vi "libssh2_trace.vi"(8 "error in (no error)":errorcluster, 10 "bitmask":i32(ring) items=["LIBSSH2_TRACE_TRANS"=2, "LIBSSH2_TRACE_KEX"=4, "LIBSSH2_TRACE_AUTH"=8, "LIBSSH2_TRACE_CONN"=16, "LIBSSH2_TRACE_SCP"=32, "LIBSSH2_TRACE_SFTP"=64, "LIBSSH2_TRACE_ERROR"=128, "LIBSSH2_TRACE_PUBLICKEY"=256, "LIBSSH2_TRACE_SOCKET"=512], 11 "session":T1) -> (0 "error out":errorcluster)   [LabVIEW 2017, in "libssh2.lvlib"]
doc: "Set the trace flags for libssh2."
uses:
  libssh2.lvlib
  Session Refnum.ctl
  Not A Session.vi
  <vilib>/Utility/error.llb/Error Cluster From Error Code.vi
  Global Settings.vi
  Read Session Refnum.vi
  <vilib>/Utility/semaphor.llb/Acquire Semaphore.vi
  <vilib>/Utility/semaphor.llb/Release Semaphore.vi
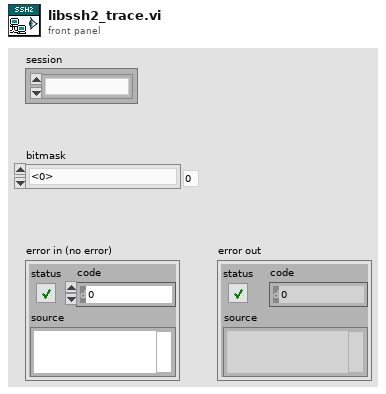
[diagram p1: front panel]
types:
  T1 = typedef "libssh2.lvlib/Session Refnum.ctl" = refnum<k1>
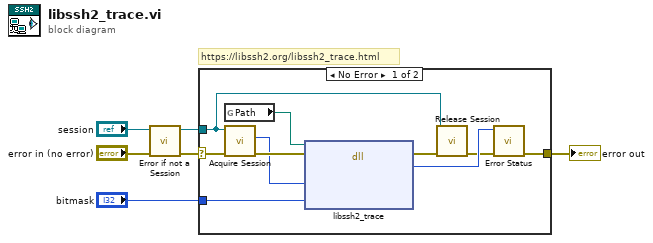
[diagram p0: block diagram]
diagram:
  # "https://libssh2.org/libssh2_trace.html"
  n1 = call "Error if not a Session.vi"("error in (no error)"="error in (no error)", "session"="session") -> ("error out"=w3:errorcluster, "session out"=w1:T1)  [unwired: 8 in]
  n2 = case shown="No Error" w3 {
    selector: w3 -> [w15 w17]
    tunnel: [w14 w17] -> w6
    tunnel: "bitmask" -> [w16 _]
    tunnel: w1 -> [w7 _]
    frame No Error {
      n3 = global read "Global Settings.vi" "Path"() -> (w10:path)
      n4 = call "Acquire Session.vi"("error in (no error)"=w15, "session"=w7) -> ("error out"=w12:errorcluster, "LIBSSH2_SESSION*"=w11:u64)  [unwired: 7 in, 1 out]
      n5 = dll-call lib="?" fn="libssh2_trace"(path in=w10, error in=w12, "session"=w11, "bitmask"=w16) -> (error out=w13:errorcluster, "return value"=w9:i32)  [unwired: 3 in, 1 out]
      n6 = call "Release Session.vi"("error in (no error)"=w13, "session"=w7) -> ("error out"=w8:errorcluster)  [unwired: 9 in]
      n7 = call "Error Status.vi"("error in (no error)"=w8, "return value"=w9) -> ("error out"=w14:errorcluster)  [unwired: 8 in, 1 out]
    }
    frame Error {
    }
  }
  "error out" <- w6
